vi "GetDropdownNamesForReport.vi"(10 "isPreSB":bool, 11 "UI 1 Data":T1={"System Log"="", "[Array Of Threshold Refs]"=[], "[Array Of Boarder Refs]"=[], "APU Type"="", "APU Setup File"={"Sensor Info"=[], "Variables"=[], "CMM Table 106"=[], "CMM Table 106B "=[], "Accel Config"=[], "Report Sheet 1"=[], "Report Sheet 2"=[], "Report Sheet 3"=[]}, "ActiveValuetoRecordRow"=[], "ReportType"=[], "ReportValue"=[], "ActiveReportSheets"=[], "APUOn"=FALSE, "APUOnTime"=timestamp(0 s since 1904-01-01), "APUOffTime"=timestamp(0 s since 1904-01-01), "Recording"=FALSE, "Test Information"={"APU Part Number:"="555", "Model:"="5", "Serial Number:"="sad", "Customer:"="sad", "Work Order:"="asd", "Pre or Post SB"="Pre SB 49-7711", "Run Count"=0, "APU Selected"="<Select>"}, "APU RUN TIME"=timestamp(0 s since 1904-01-01)} {"APU RUN TIME" format="%<%H:%M:%S>T"; "Test Information"."Run Count" min=0 step=1; "APUOffTime" format="%<%x %.3X>T"; "APUOnTime" format="%<%x %.3X>T"}) -> (2 "ActiveReportSheets":string[][](array[string]), 3 "ArraytoDIsplay":string[](array[string]))   [LabVIEW 2018, in "Testing UI 1.lvlib"]
uses:
  Testing UI 1.lvlib
  Private Controls/UI 1 Data.ctl
  Top Level/Shared Controls/APU Setup File.ctl
  File IO/Public Controls/ReportType.ctl
  Controller (Host)/Public Controls/Test Information.ctl
  Controller (Host)/Public VIs/PreorPostSB.ctl
  Controller (Host)/Public Controls/APU Select.ctl
  File IO/File IO.lvlib
  Controller (Host)/Controller (Host).lvlib
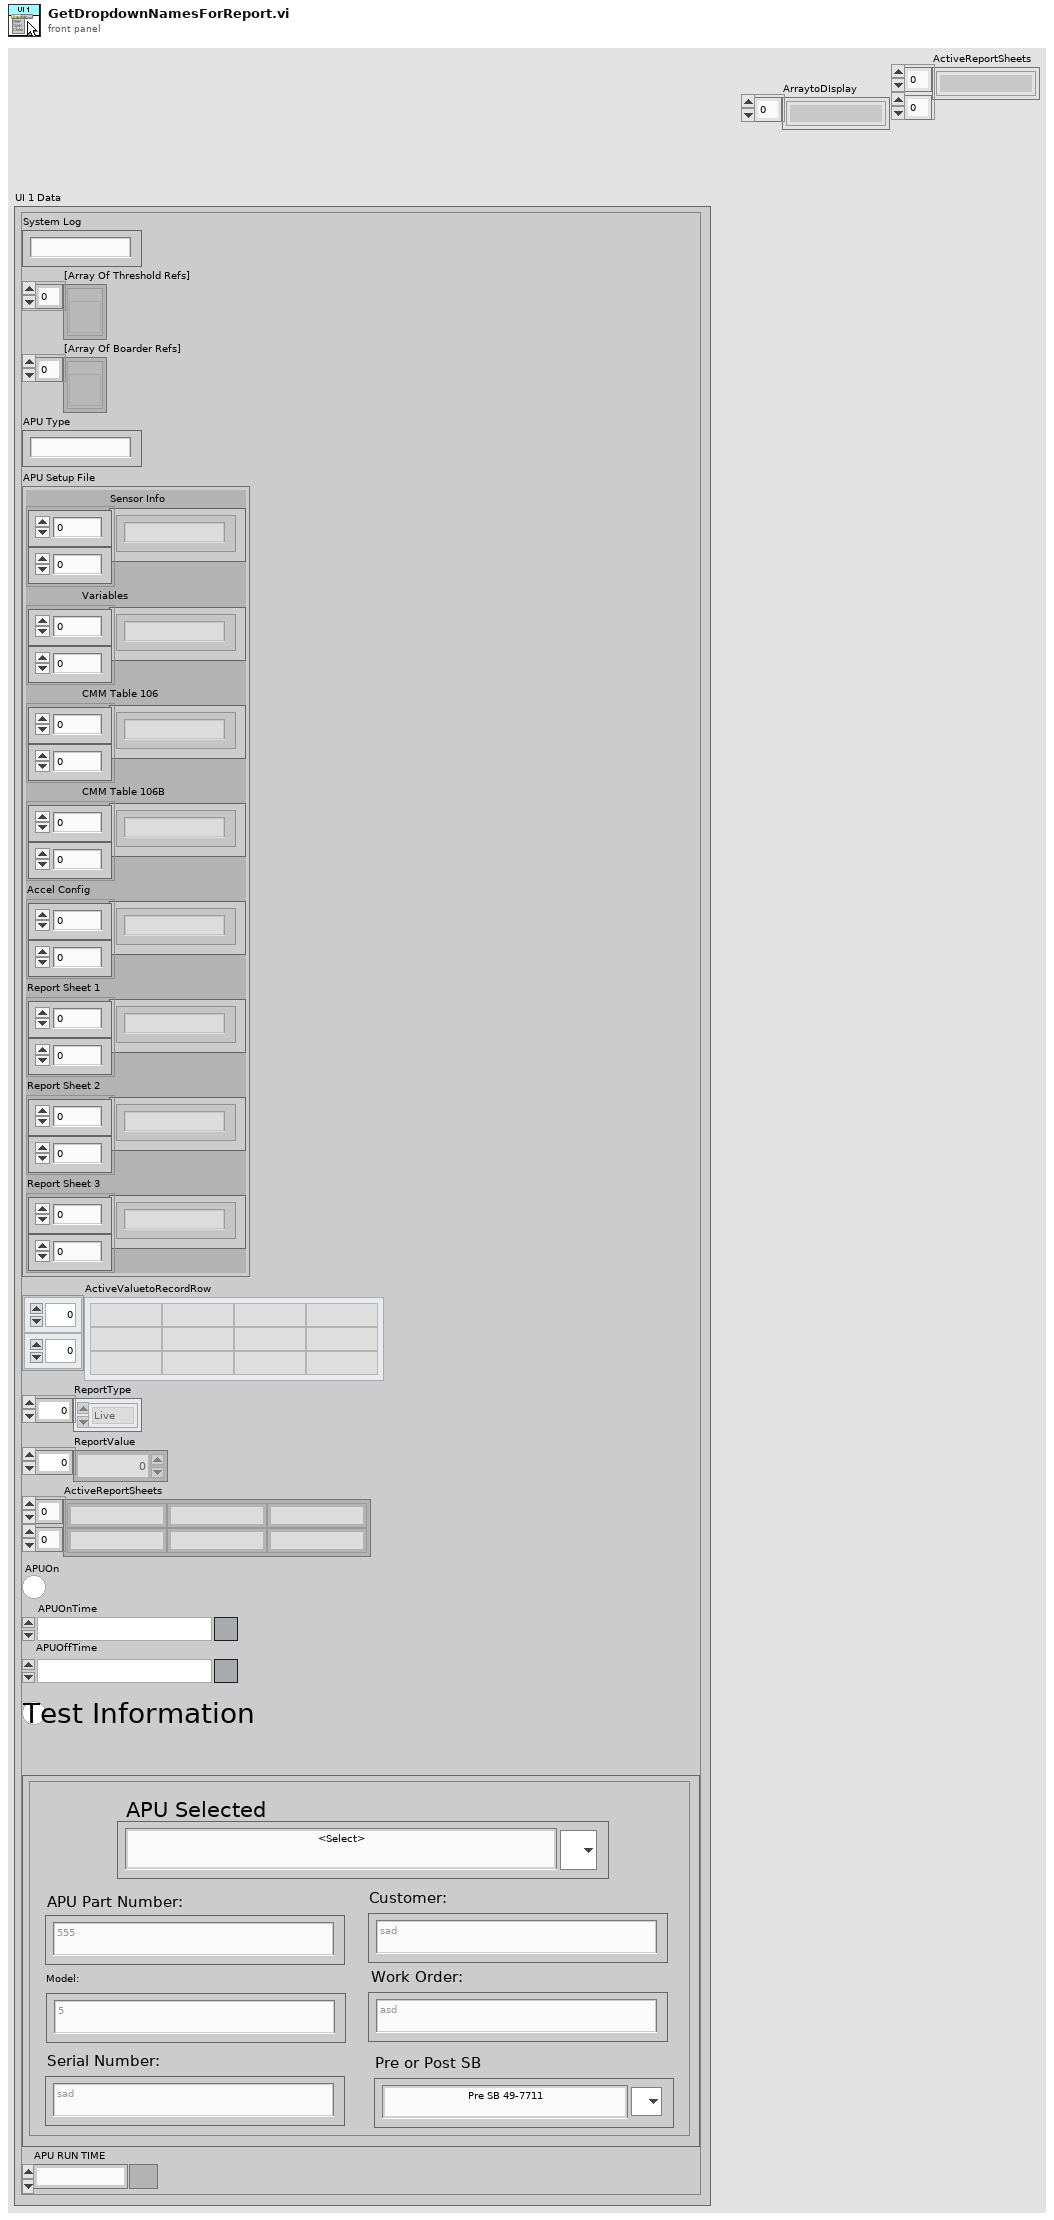
[diagram p1: front panel]
types:
  T1 = typedef "Testing UI 1.lvlib/UI 1 Data.ctl" = cluster{"System Log":string, "[Array Of Threshold Refs]":refnum<vi>[], "[Array Of Boarder Refs]":refnum<vi>[], "APU Type":string, "APU Setup File":T2, "ActiveValuetoRecordRow":string[][], "ReportType":T3[], "ReportValue":dbl[], "ActiveReportSheets":string[][], "APUOn":bool, "APUOnTime":timestamp, "APUOffTime":timestamp, "Recording":bool, "Test Information":T4, "APU RUN TIME":timestamp}
  T2 = typedef "APU Setup File.ctl" = cluster{"Sensor Info":string[][], "Variables":string[][], "CMM Table 106":string[][], "CMM Table 106B ":string[][], "Accel Config":string[][], "Report Sheet 1":string[][], "Report Sheet 2":string[][], "Report Sheet 3":string[][]}
  T3 = typedef "File IO.lvlib/ReportType.ctl" = enum16{"Live", "Min", "Max", "Deviation"}
  T4 = typedef "Controller (Host).lvlib/Test Information.ctl" = cluster{"APU Part Number:":string, "Model:":string, "Serial Number:":string, "Customer:":string, "Work Order:":string, "Pre or Post SB":T5, "Run Count":i32, "APU Selected":T6}
  T5 = typedef "Controller (Host).lvlib/PreorPostSB.ctl" = string
  T6 = typedef "Controller (Host).lvlib/APU Select.ctl" = string
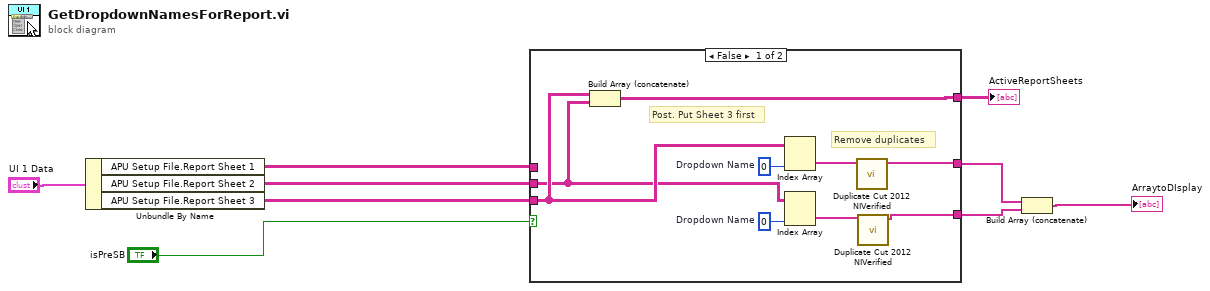
[diagram p0: block diagram]
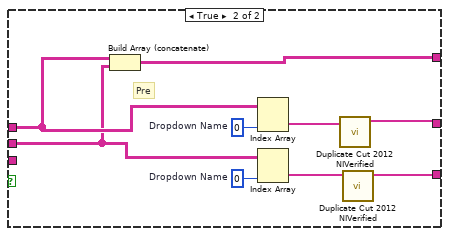
[diagram p2: hidden frame]
diagram:
  n1 = Unbundle By Name("UI 1 Data") -> ("APU Setup File.Report Sheet 1"=w2:string[][], "APU Setup File.Report Sheet 2"=w5:string[][], "APU Setup File.Report Sheet 3"=w6:string[][])
  n2 = case shown="False" "isPreSB" {
    tunnel: w2 -> [_ w21]
    tunnel: w5 -> [w11 w20]
    tunnel: w6 -> [w12 _]
    tunnel: [w15 w24] -> w7
    tunnel: [w13 w22] -> w8
    tunnel: [w10 w19] -> w1
    frame False {
      w17 = 0  # Dropdown Name
      w18 = 0  # Dropdown Name
      # "Remove duplicates"
      # "Post. Put Sheet 3 first"
      n3 = Build Array (concatenate)(w12, w11) -> (w10:string[][])
      n4 = Index Array(array=w12, index (col)=w18) -> (element=w16:string[])  [unwired: 1 in]
      n5 = Index Array(array=w11, index (col)=w17) -> (element=w14:string[])  [unwired: 1 in]
      n6 = call "Duplicate Cut 2012 NIVerified.vi"("Array In"=w16) -> ("Array Out"=w15:string[])  [unwired: 10 in]
      n7 = call "Duplicate Cut 2012 NIVerified.vi"("Array In"=w14) -> ("Array Out"=w13:string[])  [unwired: 10 in]
    }
    frame True {
      w26 = 0  # Dropdown Name
      w27 = 0  # Dropdown Name
      # "Pre"
      n8 = Build Array (concatenate)(w21, w20) -> (w19:string[][])
      n9 = Index Array(array=w21, index (col)=w27) -> (element=w25:string[])  [unwired: 1 in]
      n10 = Index Array(array=w20, index (col)=w26) -> (element=w23:string[])  [unwired: 1 in]
      n11 = call "Duplicate Cut 2012 NIVerified.vi"("Array In"=w25) -> ("Array Out"=w24:string[])  [unwired: 10 in]
      n12 = call "Duplicate Cut 2012 NIVerified.vi"("Array In"=w23) -> ("Array Out"=w22:string[])  [unwired: 10 in]
    }
  }
  "ActiveReportSheets" <- w1
  n13 = Build Array (concatenate)(w7, w8) -> (→"ArraytoDIsplay":string[])
